vi "TEST.vi"() -> ()   [LabVIEW 2016]
uses:
  interface.vi
  Alarm interface.lvlib
panel:
  in  "退出":bool
  in  "报警接口":bool
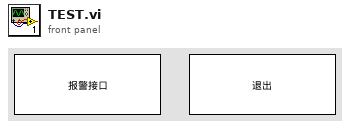
[diagram p1: front panel]
types:
  T1 = enum32{"Invalid", "Standard", "Closed", "Hidden", "Minimized", "Maximized"}
  T2 = enum32{"Bad", "Idle", "Run top level", "Running"}
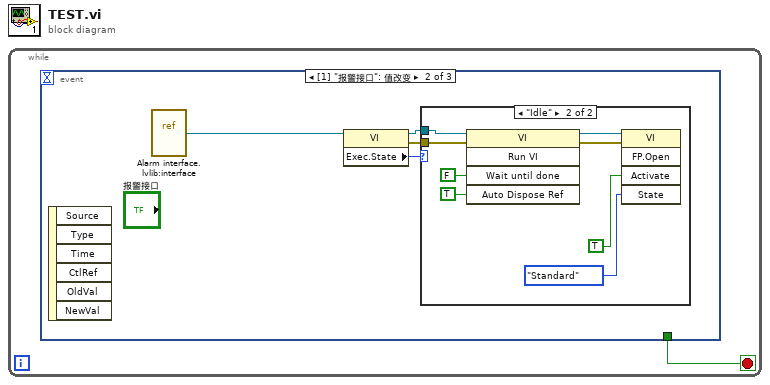
[diagram p0: block diagram]
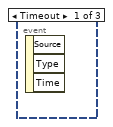
[diagram p2: hidden frame]
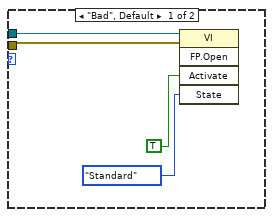
[diagram p3: hidden frame]
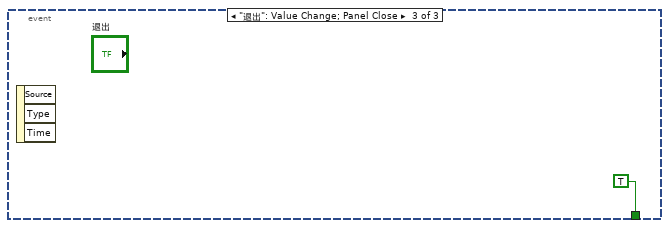
[diagram p4: hidden frame]
diagram:
  n1 = while {
    stop <- w1 stop-if-true
    n2 = event shown="[1] \"报警接口\": 值改变" {
      selector: _ -> [_ _ _]
      dyn-events: _ -> [_ _ _]
      timeout: _ -> [_ _ _]
      tunnel: [_ _ TRUE] -> w1
      event Timeout {
        n3 = event-data() -> ()  [unwired: 1 in, 3 out]
      }
      event "报警接口": Value Change {
        n4 = event-data() -> ()  [unwired: 1 in, 6 out]
        n5 = vi-ref "Alarm interface.lvlib:interface.vi"() -> (w3:refnum<vi>)
        n6 = property class="VI"(reference=w3) -> (reference out=w4:refnum<vi>, error out=w2:errorcluster, "Exec.State"=w5:T2)  [unwired: 1 in]
        n7 = case shown="\"Idle\"" w5 {
          tunnel: w4 -> [w7 w15]
          tunnel: w2 -> [w6 w13]
          frame "Bad", Default {
            n8 = invoke class="VI" method="FP.Open"(reference=w7, error in=w6, "Activate"=TRUE ("激活？"), "State"=T1."Standard" ("状态")) -> ()  [unwired: 1 in, 5 out]
          }
          frame "Idle" {
            n9 = invoke class="VI" method="Run VI"(reference=w15, error in=w13, "Wait until done"=FALSE ("结束前等待"), "Auto Dispose Ref"=TRUE ("自动销毁引用")) -> (reference out=w14:refnum<vi>, error out=w12:errorcluster)  [unwired: 1 in, 3 out]
            n10 = invoke class="VI" method="FP.Open"(reference=w14, error in=w12, "Activate"=TRUE ("激活？"), "State"=T1."Standard" ("状态")) -> ()  [unwired: 1 in, 5 out]
          }
        }
      }
      event "退出": Value Change; Panel Close {
        n11 = event-data() -> ()  [unwired: 1 in, 3 out]
      }
    }
  }
